vi "Z_Meas_Gate.vi"(8 "error in (no error)":errorcluster, 11 "QuWire in":refnum<class "QuWire.lvclass">) -> (0 "error out":errorcluster, 2 "Classical bit":bool, 3 "QuWire out":refnum<class "QuWire.lvclass">)   [LabVIEW 2020, in "QuWire.lvclass"]
uses:
  QuWire.lvclass
  QuWire.lvclass/QuWire.ctl
  SimAlg/PrllPerElement/PrllPerElmnt.lvclass
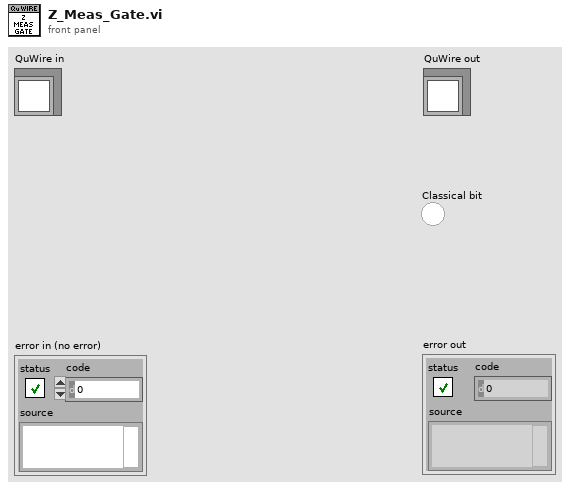
[diagram p1: front panel]
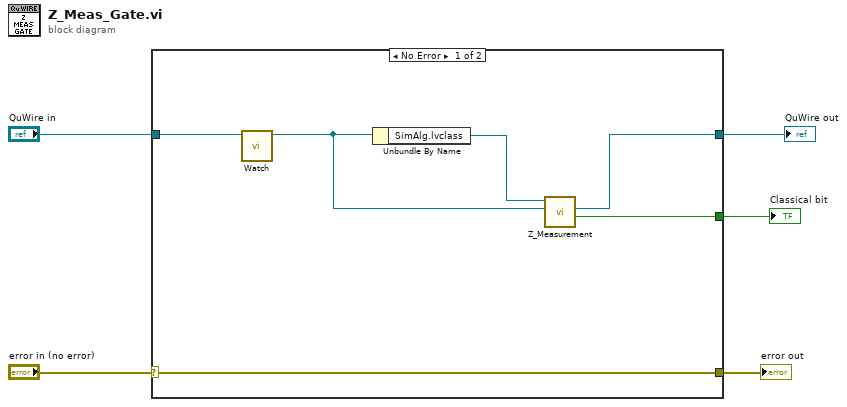
[diagram p0: block diagram]
diagram:
  n1 = case shown="No Error" "error in (no error)" {
    selector: "error in (no error)" -> [w11 w13]
    tunnel: [w11 w13] -> w4
    tunnel: "QuWire in" -> [w10 w12]
    tunnel: [w9 _] -> w2
    tunnel: [w8 w12] -> w1
    frame No Error {
      n2 = call "Watch.vi"("QuWire in"=w10) -> ("QuWire out"=w6:refnum<class "QuWire.lvclass">)  [unwired: 9 in, 1 out]
      n3 = Unbundle By Name(w6) -> ("SimAlg.lvclass"=w7:refnum<class "PrllPerElmnt.lvclass">)
      n4 = call-dynamic "Z_Measurement.vi"("QuWire in"=w6, "SimAlg in"=w7) -> ("Classical bit"=w9:bool, "QuWire out"=w8:refnum<class "QuWire.lvclass">)  [unwired: 6 in, 2 out]
    }
    frame Error {
    }
  }
  "error out" <- w4
  "Classical bit" <- w2
  "QuWire out" <- w1
